vi "SQLDriverConnect.vi"(4 "Password":string, 5 "error in (no error)":errorcluster, 6 "UserName":string, 7 "Database Path (empty)":path, 8 "InputHandle":i32) -> (0 "error out":errorcluster, 2 "ConnectionString":string, 3 "OutputHandle":i32)   [LabVIEW 2011]
doc: "Se connecte auprès de la base spécifiée. S'identifie par le nom d'utilisateur et le mot de passe associé"
uses:
  Odbc32.dll
panel:
  out "OutConnectionString":string
  out "Overflow":i16
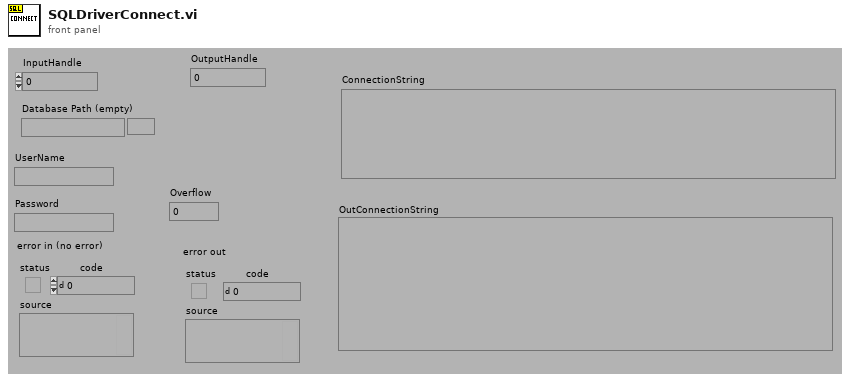
[diagram p1: front panel]
types:
  T1 = enum16{"NOPE", "SQL_HANDLE_ENV", "SQL_HANDLE_DBC", "SQL_HANDLE_STMT", "SQL_HANDLE_DESC"}
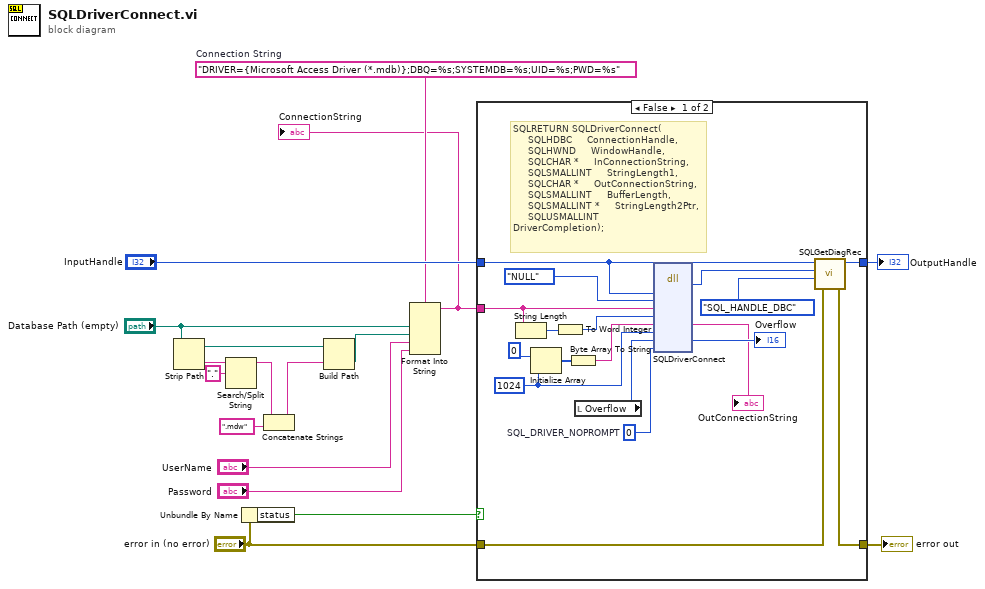
[diagram p0: block diagram]
diagram:
  w12 = "DRIVER={Microsoft Access Driver (*.mdb)};DBQ=%s;SYSTEMDB=%s;UID=%s;PWD=%s"  # Connection String
  n1 = Strip Path(path="Database Path (empty)") -> (stripped path=w8:path, name=w7:string)
  n2 = Search/Split String(string=w7, search string/char (-)=".") -> (substring before match=w5:string)  [unwired: 3 out]
  n3 = Unbundle By Name("error in (no error)") -> ("status"=w16:bool)
  n4 = Concatenate Strings(w5, ".mdw" ("string")) -> (w3:string)
  n5 = Build Path(base path=w8, name or relative path=w3) -> (appended path=w1:path)
  n6 = Format Into String(format string=w12, "Database Path (empty)", w1, "UserName", "Password") -> (resulting string=w2:string)  [unwired: 2 in, 1 out]
  "ConnectionString" <- w2
  n7 = case shown="False" w16 {
    tunnel: "InputHandle" -> [w35 w37]
    tunnel: "error in (no error)" -> [w33 w36]
    tunnel: [w32 w36] -> w15
    tunnel: [w34 w37] -> w14
    tunnel: w2 -> [w20 _]
    frame False {
      w23 = u16 0  # SQL_DRIVER_NOPROMPT
      w24 = i16 1024 ("dimension size")
      # "SQLRETURN SQLDriverConnect(\n     SQLHDBC     ConnectionHandle,\n     SQLHWND     WindowHandle,\n     SQLCHAR *     InConnectionString,\n     SQLSMALLINT     StringLength1,\n     SQLCHAR *     OutConnectionString,\n     SQLSMALLINT     BufferLength,\n     SQLSMALLINT *     StringLength2Ptr,\n     SQLUSMALLINT     DriverCompletion);"
      n8 = String Length(string=w20) -> (length=w28:i32)
      n9 = Initialize Array(u8 0, w24) -> (w25:u8[])
      n10 = To Word Integer(number=w28) -> (16bit integer=w27:i16)
      n11 = Byte Array To String(unsigned byte array=w25) -> (string=w18:string)
      n12 = local read "Overflow"() -> (w22:i16)
      n13 = dll-call lib="Odbc32.dll" fn="SQLDriverConnect"("ConnectionHandle"=w35, "WindowHandle"=enum32{"NULL"}."NULL", "InConnectionString"=w20, "StringLength1"=w27, "OutConnectionString"=w18, "BufferLength"=w24, "StringLength2Ptr"=w22, "DriverCompletion"=w23) -> ("SQLRETURN"=w31:i16, "OutConnectionString"=→"OutConnectionString":string, "StringLength2Ptr"=→"Overflow":i16)  [unwired: 8 in, 3 out]
      n14 = call "SQLGetDiagRec.vi"("error in (no error)"=w33, "HandleType"=T1."SQL_HANDLE_DBC", "Status (SQL_SUCCESS=0)"=w31, "Input Handle"=w35) -> ("error out"=w32:errorcluster, "Output Handle"=w34:i32)  [unwired: 2 out]
    }
    frame True {
    }
  }
  "OutputHandle" <- w14
  "error out" <- w15
